vi "Convert Step to String.vi"(11 "Step":T1) -> (3 "Step String":string)   [LabVIEW 2020, in "MacroAssert.lvlib"]
uses:
  MacroAssert.lvlib
  CTLs/Step Type V3.ctl
  CTLs/Assertion Type.ctl
  CTLs/Step V3.ctl
  <vilib>/picture/picture.llb/imagedata.ctl
panel:
  in  "Virtual Key":u8(ring)=65
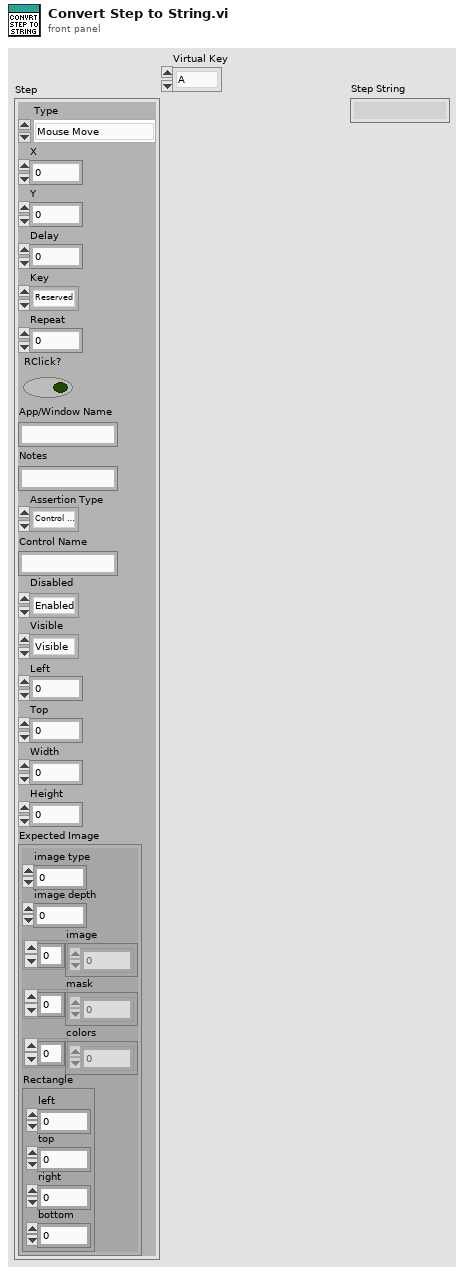
[diagram p1: front panel]
types:
  T1 = typedef "MacroAssert.lvlib/Step V3.ctl" = cluster{"Type":T2, "X":i32, "Y":i32, "Delay":i32, "Key":u8, "Repeat":i32, "RClick?":bool, "App/Window Name":string, "Notes":string, "Assertion Type":T3, "Control Name":string, "Disabled":enum8{"Enabled", "Disabled", "Disabled and Grayed Out"}, "Visible":enum16{"Visible", "Not Visible"}, "Left":i16, "Top":i16, "Width":i16, "Height":i16, "Expected Image":T4}
  T2 = typedef "MacroAssert.lvlib/Step Type V3.ctl" = enum16{"Mouse Move", "Mouse Click", "Key Press", "Wait", "Mouse Down", "Mouse Up", "Key Down", "Key Up", "Test Assertion", "Run Application", "Maximize Window", "Restore Window", "Minimize Window", "Close Window", "Bring Window to Front", "Send Window to Back"}
  T3 = typedef "MacroAssert.lvlib/Assertion Type.ctl" = enum16{"Control Position", "Control Visible", "Control Disabled", "Control Image"}
  T4 = typedef "imagedata.ctl" = cluster{"image type":i32, "image depth":i32, "image":u8[], "mask":u8[], "colors":u32[], "Rectangle":cluster{"left":i16, "top":i16, "right":i16, "bottom":i16}}
  T5 = enum8{"Enabled", "Disabled", "Disabled and Grayed Out"}
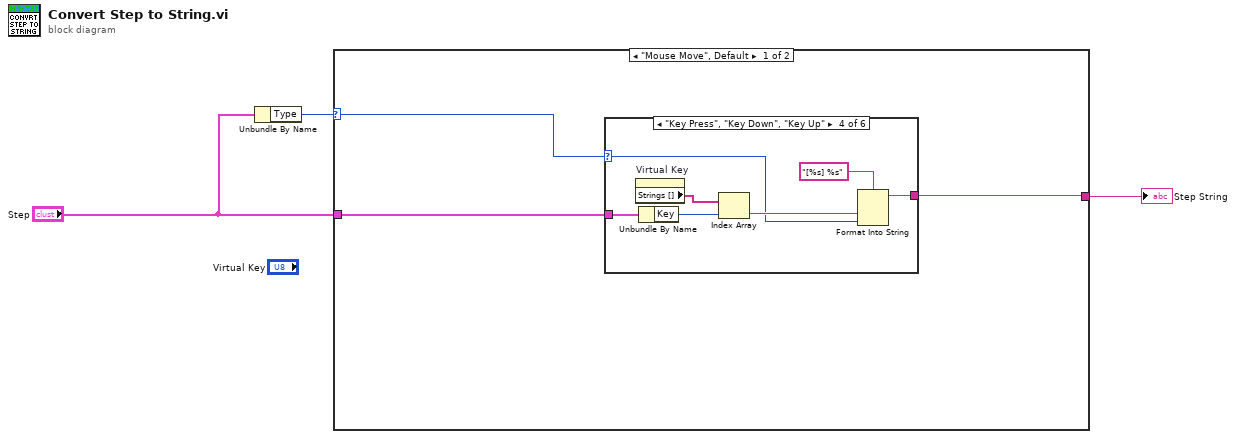
[diagram p0: block diagram]
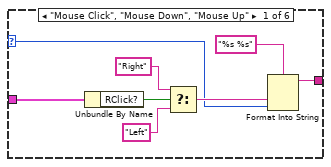
[diagram p2: hidden frame]
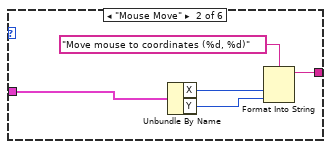
[diagram p3: hidden frame]
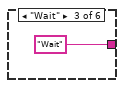
[diagram p4: hidden frame]
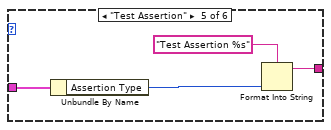
[diagram p5: hidden frame]
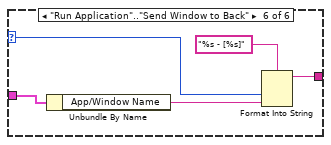
[diagram p6: hidden frame]
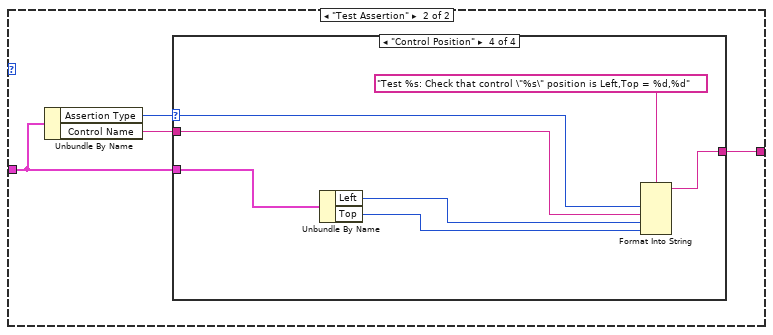
[diagram p7: hidden frame]
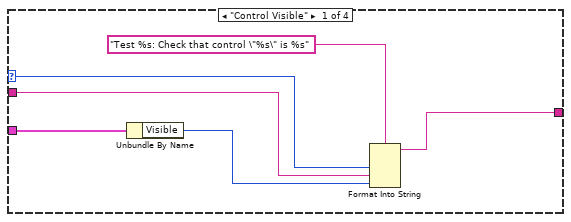
[diagram p8: hidden frame]
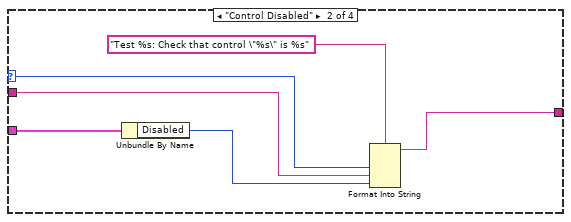
[diagram p9: hidden frame]
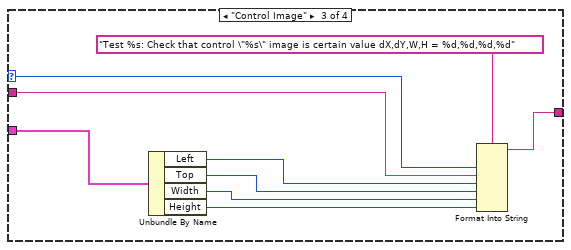
[diagram p10: hidden frame]
diagram:
  n1 = Unbundle By Name("Step") -> ("Type"=w3:T2)
  n2 = case shown="\"Mouse Move\", Default" w3 {
    selector: w3 -> [w6 _]
    tunnel: "Step" -> [w5 w38]
    tunnel: [w4 w39] -> w1
    frame "Mouse Move", Default {
      n3 = case shown="\"Key Press\", \"Key Down\", \"Key Up\"" w6 {
        selector: w6 -> [w8 _ _ w22 _ w34]
        tunnel: w5 -> [w10 w19 _ w27 w31 w36]
        tunnel: [w7 w18 "Wait" w21 w29 w33] -> w4
        frame "Mouse Click", "Mouse Down", "Mouse Up" {
          n4 = Unbundle By Name(w10) -> ("RClick?"=w13:bool)
          n5 = Select(t="Right", s=w13, f="Left") -> (s? t:f=w9:string)
          n6 = Format Into String(format string="%s %s", w9, w8) -> (resulting string=w7:string)  [unwired: 2 in, 1 out]
        }
        frame "Mouse Move" {
          n7 = Unbundle By Name(w19) -> ("X"=w16:i32, "Y"=w15:i32)
          n8 = Format Into String(format string="Move mouse to coordinates (%d, %d)", w16, w15) -> (resulting string=w18:string)  [unwired: 2 in, 1 out]
        }
        frame "Wait" {
        }
        frame "Key Press", "Key Down", "Key Up" {
          n9 = property on="Virtual Key" class="Ring (strict)"() -> ("Strings []"=w25:string[])  [unwired: 2 in, 2 out]
          n10 = Unbundle By Name(w27) -> ("Key"=w24:u8)
          n11 = Index Array(array=w25, index=w24) -> (element=w23:string)
          n12 = Format Into String(format string="[%s] %s", w23, w22) -> (resulting string=w21:string)  [unwired: 2 in, 1 out]
        }
        frame "Test Assertion" {
          n13 = Unbundle By Name(w31) -> ("Assertion Type"=w28:T3)
          n14 = Format Into String(format string="Test Assertion %s", w28) -> (resulting string=w29:string)  [unwired: 2 in, 1 out]
        }
        frame "Run Application".."Send Window to Back" {
          n15 = Unbundle By Name(w36) -> ("App/Window Name"=w32:string)
          n16 = Format Into String(format string="%s - [%s]", w34, w32) -> (resulting string=w33:string)  [unwired: 2 in, 1 out]
        }
      }
    }
    frame "Test Assertion" {
      n17 = Unbundle By Name(w38) -> ("Assertion Type"=w40:T3, "Control Name"=w37:string)
      n18 = case shown="\"Control Position\"" w40 {
        selector: w40 -> [w45 w51 w60 w67]
        tunnel: [w44 w50 w59 w66] -> w39
        tunnel: w38 -> [w42 w48 w57 w64]
        tunnel: w37 -> [w43 w49 w58 w65]
        frame "Control Visible" {
          n19 = Unbundle By Name(w42) -> ("Visible"=w41:enum16{"Visible", "Not Visible"})
          n20 = Format Into String(format string="Test %s: Check that control \"%s\" is %s", w45, w43, w41) -> (resulting string=w44:string)  [unwired: 2 in, 1 out]
        }
        frame "Control Disabled" {
          n21 = Unbundle By Name(w48) -> ("Disabled"=w47:T5)
          n22 = Format Into String(format string="Test %s: Check that control \"%s\" is %s", w51, w49, w47) -> (resulting string=w50:string)  [unwired: 2 in, 1 out]
        }
        frame "Control Image" {
          n23 = Unbundle By Name(w57) -> ("Left"=w53:i16, "Top"=w54:i16, "Width"=w55:i16, "Height"=w56:i16)
          n24 = Format Into String(format string="Test %s: Check that control \"%s\" image is certain value dX,dY,W,H = %d,%d,%d,%d", w60, w58, w53, w54, w55, w56) -> (resulting string=w59:string)  [unwired: 2 in, 1 out]
        }
        frame "Control Position" {
          n25 = Unbundle By Name(w64) -> ("Left"=w62:i16, "Top"=w63:i16)
          n26 = Format Into String(format string="Test %s: Check that control \"%s\" position is Left,Top = %d,%d", w67, w65, w62, w63) -> (resulting string=w66:string)  [unwired: 2 in, 1 out]
        }
      }
    }
  }
  "Step String" <- w1
